vi "Actor Core.vi"(8 "error in":errorcluster, 11 "Nested in":refnum<class "  SEÑAL_ACTUALIZABLE.lvclass">) -> (0 "error out":errorcluster, 3 "Actor out":refnum<class "Actor.lvclass">)   [LabVIEW 2019, in "  SEÑAL_ACTUALIZABLE.lvlib" / "  SEÑAL_ACTUALIZABLE.lvclass"]
doc: "(<B>Filename</B>: Actor Framework.lvlib:Actor.lvclass:Actor Core.vi)\n\nReceives messages to the actor, reacts to them, and initiates any error handling that may shut the actor down.\n\nDescendant classes may override this VI to append parallel tasks for the actor to complete while it handles messages. Overrides use the Call Parent Method node."
uses:
  C:/Program Files (x86)/National Instruments/LabVIEW 2019/vi.lib/ActorFramework/Actor/Actor.lvclass
  <vilib>/ActorFramework/Actor/Actor.lvclass
  GUARDADOTEXTOPLANO/GUARDADOTEXTOPLANO/GUARDADOTEXTOPLANO.lvclass
  <vilib>/ActorFramework/Actor/Actor.lvclass/Actor.ctl
  <vilib>/ActorFramework/Message Enqueuer/Message Enqueuer.lvclass/Message Enqueuer.ctl
  GUARDADOTEXTOPLANO/GUARDADOTEXTOPLANO Messages/SEND_INICIARG Msg/SEND_INICIARG Msg.lvclass/SEND_INICIARG Msg.ctl
  GUARDADOTEXTOPLANO/GUARDADOTEXTOPLANO Messages/DATOS Y GUARDADO Msg/DATOS Y GUARDADO Msg.lvclass/DATOS Y GUARDADO Msg.ctl
  <vilib>/ActorFramework/Message Enqueuer/Init from Existing Queue.vi
  <vilib>/ActorFramework/Message Enqueuer/Enqueue.vi
  <vilib>/ActorFramework/Stop Msg/Stop Msg.lvclass
  C:/Program Files (x86)/National Instruments/LabVIEW 2019/vi.lib/ActorFramework/Message/Message.lvclass
  GUARDADOTEXTOPLANO/GUARDADOTEXTOPLANO Messages/SEND_INICIARG Msg/SEND_INICIARG Msg.lvclass
  GUARDADOTEXTOPLANO/GUARDADOTEXTOPLANO Messages/DATOS Y GUARDADO Msg/DATOS Y GUARDADO Msg.lvclass
  <vilib>/ActorFramework/Message Priority Queue/Priority Enqueue.vi
  <vilib>/ActorFramework/Message Enqueuer/Message Enqueuer.lvclass
panel:
  out "Waveform Graph":waveform(dbl)(graph)
  in  "GUARDAR":bool
  in  "Path 2":path
  in  "Parámetros":T1={"signal type"=enum."Sine Wave", "amplitude"=1.0, "frequency"=10.0} {"frequency" format="%0.2p"; "amplitude" format="%0.2p"}
  in  "EXIT":bool
  in  "STOP":bool
  in  "START":bool
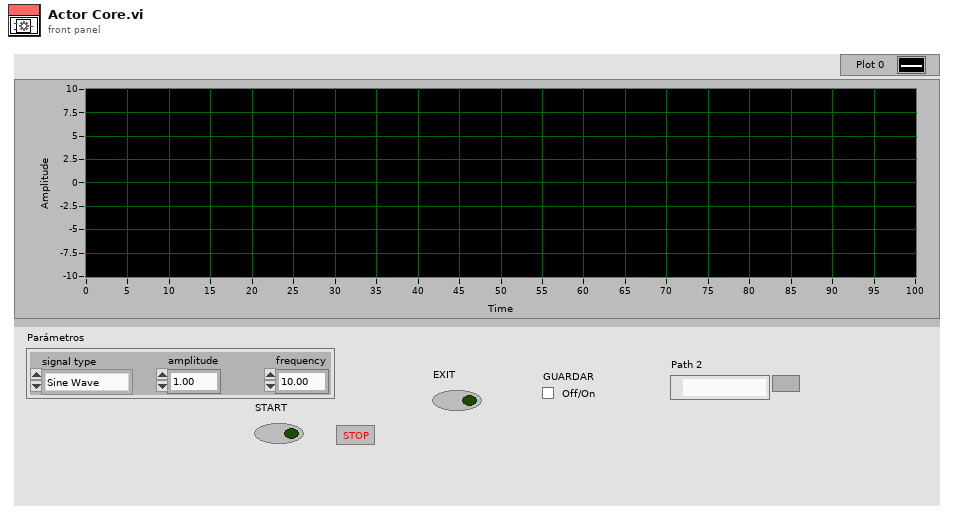
[diagram p1: front panel]
types:
  T1 = cluster{"signal type":enum16{"Sine Wave", "Triangle Wave", "Square Wave", "Sawtooth Wave"}, "amplitude":dbl, "frequency":dbl}
  T2 = cluster{"Stop":refnum<user-event>, "Waveform Graph":refnum<user-event>}
  T3 = enum16{"Sine Wave", "Triangle Wave", "Square Wave", "Sawtooth Wave"}
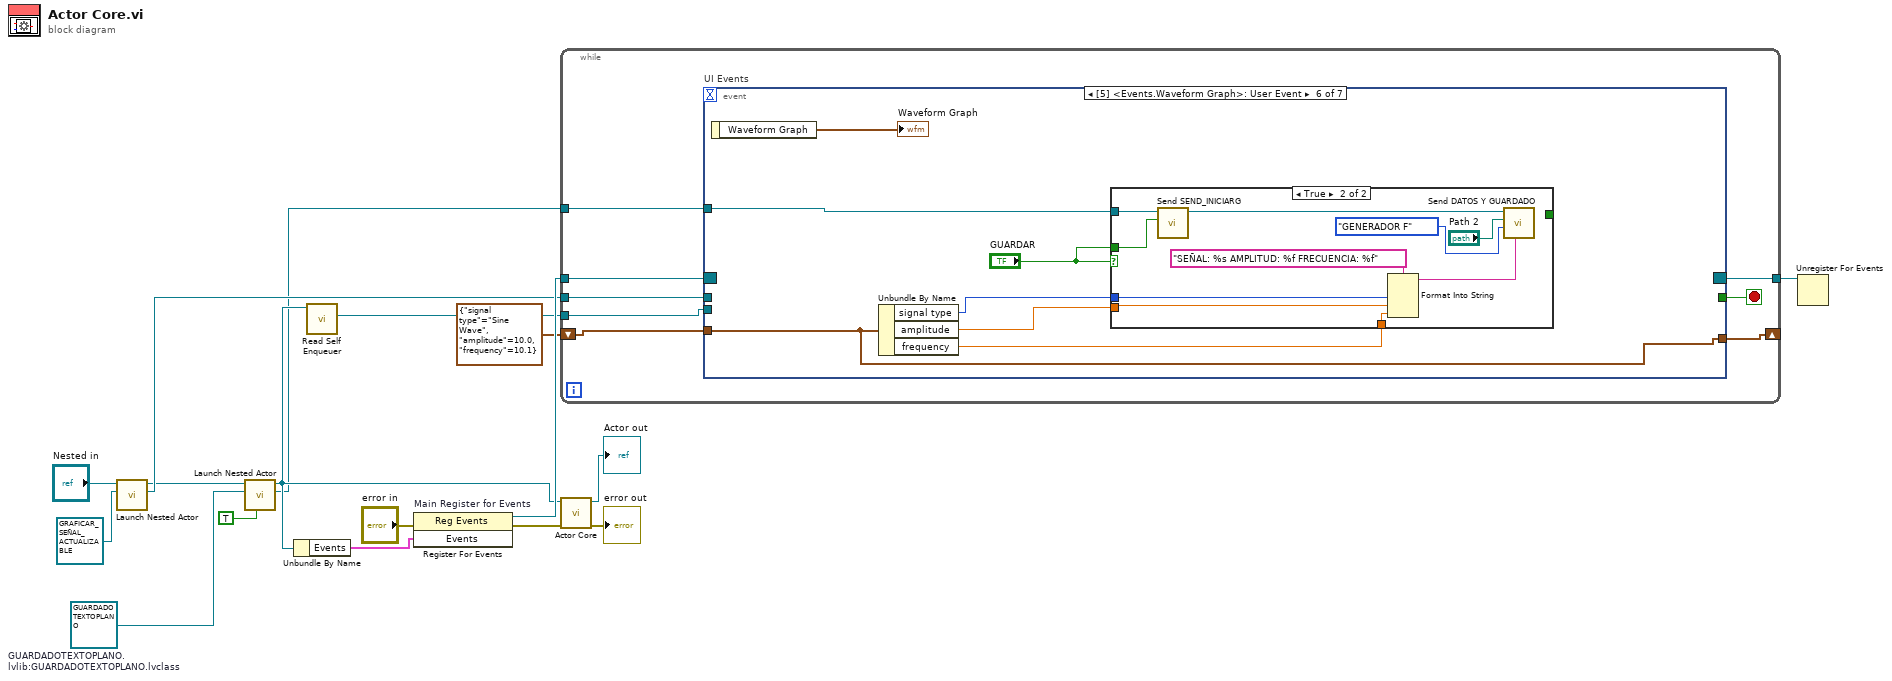
[diagram p0: block diagram]
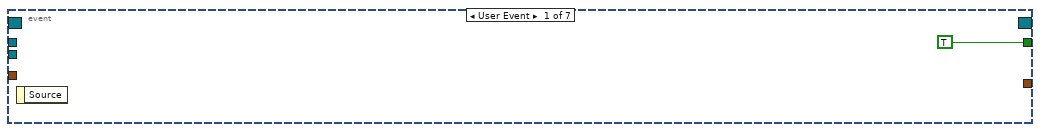
[diagram p2: hidden frame]
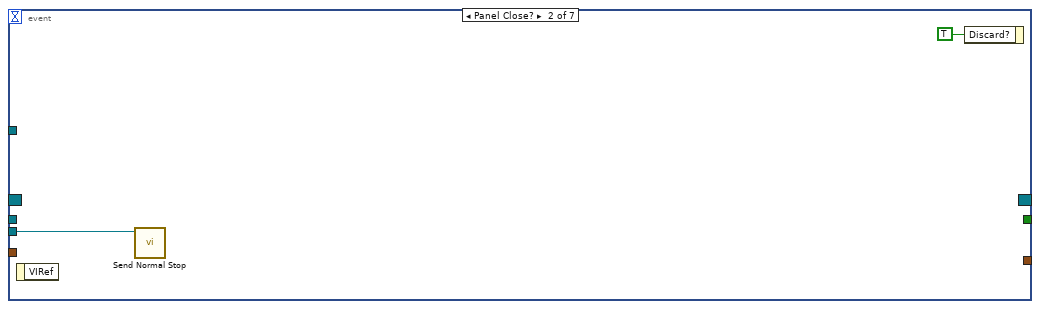
[diagram p3: hidden frame]
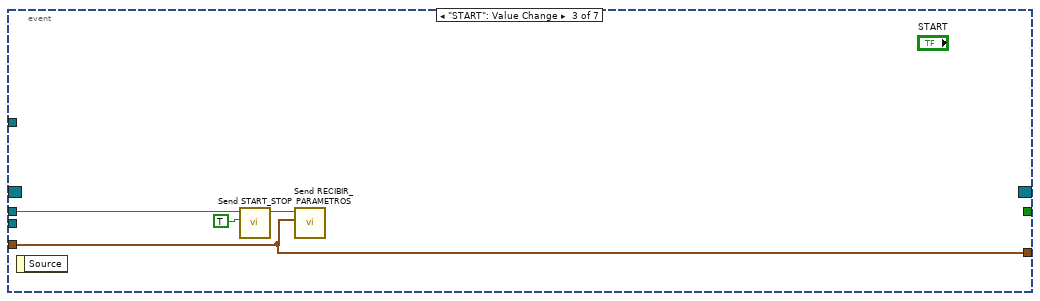
[diagram p4: hidden frame]
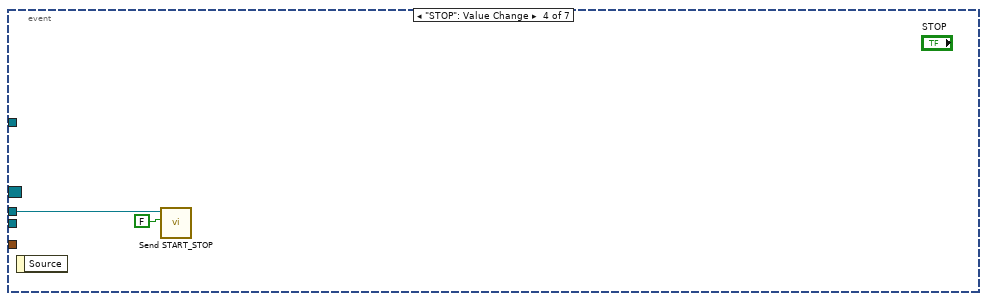
[diagram p5: hidden frame]
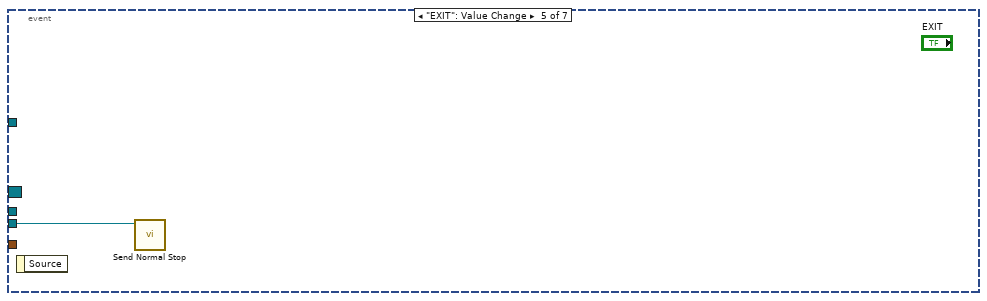
[diagram p6: hidden frame]
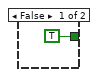
[diagram p7: hidden frame]
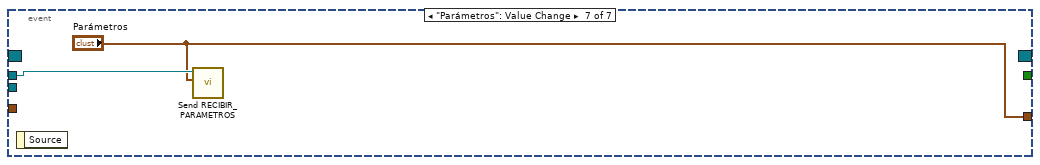
[diagram p8: hidden frame]
diagram:
  w6 = refnum<class "GUARDADOTEXTOPLANO.lvclass"> refnum  # GUARDADOTEXTOPLANO.lvlib:GUARDADOTEXTOPLANO.lvclass
  n1 = call <vilib>:"Launch Nested Actor.vi"("Nested Actor"=refnum<class "GRAFICAR_SEÑAL_ACTUALIZABLE.lvclass"> refnum ("GRAFICAR_SEÑAL_ACTUALIZABLE.lvlib:GRAFICAR_SEÑAL_ACTUALIZABLE.lvclass"), "Caller Actor in"="Nested in") -> ("Nested Actor's Enqueuer"=w8:refnum<class "Message Enqueuer.lvclass">, "Caller Actor out"=w5:refnum<class "  SEÑAL_ACTUALIZABLE.lvclass">)  [unwired: 7 in, 1 out]
  n2 = call <vilib>:"Launch Nested Actor.vi"("Open Actor Core front panel? (F)"=TRUE, "Nested Actor"=w6, "Caller Actor in"=w5) -> ("Nested Actor's Enqueuer"=w3:refnum<class "Message Enqueuer.lvclass">, "Caller Actor out"=w4:refnum<class "  SEÑAL_ACTUALIZABLE.lvclass">)  [unwired: 6 in, 1 out]
  n3 = Unbundle By Name(w4) -> ("Events"=w14:T2)
  n4 = call <vilib>:"Read Self Enqueuer.vi"("Actor"=w4) -> ("Self Enqueuer"=w12:refnum<class "Message Enqueuer.lvclass">)  [unwired: 10 in]
  n5 = register-events "Main Register for Events"(error in="error in", w14) -> (reference out=w15:refnum<event-registration>, error out=w10:errorcluster)  [unwired: 1 in]
  n6 = while {
    tunnel: w15 -> [w25]
    tunnel: [w23] -> w13
    tunnel: w12 -> [w22]
    tunnel: w8 -> [w21]
    tunnel: w3 -> [w20]
    shift-right: [w18] -> _
    shift-left: T1 {"signal type"=enum."Sine Wave", "amplitude"=10.0, "frequency"=10.1} ("Parámetros") -> [w19]
    stop <- w24 stop-if-true
    n7 = event "UI Events" shown="[5] <Events.Waveform Graph>: User Event" {
      selector: w25 -> [_ _ _ _ _ _ _]
      dyn-events: [_ _ _ _ _ _ _] -> w23
      timeout: _ -> [_ _ _ _ _ _ _]
      tunnel: [TRUE _ _ _ _ _ _] -> w24
      tunnel: w22 -> [_ w27 _ _ w35 _ _]
      tunnel: w21 -> [_ _ w32 w34 _ _ w55]
      tunnel: w20 -> [_ _ _ _ _ w42 _]
      tunnel: w19 -> [_ _ w29 _ _ w36 _]
      tunnel: [_ _ w29 _ _ w36 "Parámetros"] -> w18
      event User Event {
        n8 = event-data() -> ()  [unwired: 1 in, 1 out]
      }
      event Panel Close? {
        n9 = event-data() -> ()  [unwired: 1 in, 1 out]
        n10 = call <vilib>:"Send Normal Stop.vi"("Message Enqueuer"=w27) -> ()  [unwired: 10 in, 1 out]
        n11 = event-data("Discard?"=TRUE) -> ()  [unwired: 1 in, 1 out]
      }
      event "START": Value Change {
        n12 = event-data() -> ()  [unwired: 1 in, 1 out]
        n13 = call "Send START_STOP.vi"("START/STOP"=TRUE, "Message Enqueuer"=w32) -> ("Message Enqueuer out"=w30:refnum<class "Message Enqueuer.lvclass">)  [unwired: 8 in, 1 out]
        n14 = call "Send RECIBIR_PARAMETROS.vi"("Parámetros"=w29, "Message Enqueuer"=w30) -> ()  [unwired: 8 in, 2 out]
      }
      event "STOP": Value Change {
        n15 = event-data() -> ()  [unwired: 1 in, 1 out]
        n16 = call "Send START_STOP.vi"("START/STOP"=FALSE, "Message Enqueuer"=w34) -> ()  [unwired: 8 in, 2 out]
      }
      event "EXIT": Value Change {
        n17 = event-data() -> ()  [unwired: 1 in, 1 out]
        n18 = call <vilib>:"Send Normal Stop.vi"("Message Enqueuer"=w35) -> ()  [unwired: 10 in, 1 out]
      }
      event User Event {
        n19 = event-data() -> ("Waveform Graph"=→"Waveform Graph":waveform(dbl))  [unwired: 1 in]
        n20 = Unbundle By Name(w36) -> ("signal type"=w39:T3, "amplitude"=w38:dbl, "frequency"=w37:dbl)
        n21 = case shown="True" "GUARDAR" {
          tunnel: "GUARDAR" -> [_ w53]
          tunnel: w42 -> [_ w49]
          tunnel: [TRUE _] -> _
          tunnel: w39 -> [_ w46]
          tunnel: w38 -> [_ w45]
          tunnel: w37 -> [_ w44]
          frame False {
          }
          frame True {
            n22 = call "Send SEND_INICIARG.vi"("GUARDAR?"=w53, "Message Enqueuer"=w49) -> ("Message Enqueuer out"=w52:refnum<class "Message Enqueuer.lvclass">)  [unwired: 8 in, 1 out]
            n23 = Format Into String(format string="SEÑAL: %s AMPLITUD: %f FRECUENCIA: %f", w46, w45, w44) -> (resulting string=w48:string)  [unwired: 2 in, 1 out]
            n24 = call "Send DATOS Y GUARDADO.vi"("DATO"=w48, "PROVIENE DE?"=enum16{"CONTADOR", "GENERADOR F"}."GENERADOR F", "Path"="Path 2", "Message Enqueuer"=w52) -> ()  [unwired: 6 in, 2 out]
          }
        }
      }
      event "Parámetros": Value Change {
        n25 = event-data() -> ()  [unwired: 1 in, 1 out]
        n26 = call "Send RECIBIR_PARAMETROS.vi"("Parámetros"="Parámetros", "Message Enqueuer"=w55) -> ()  [unwired: 8 in, 2 out]
      }
    }
  }
  n27 = call-parent "Actor Core.vi"("error in"=w10, "Actor in"=w4) -> ("error out"=→"error out":errorcluster, "Actor out"=→"Actor out":refnum<class "Actor.lvclass">)  [unwired: 8 in]
  n28 = Unregister For Events(event registration refnum=w13) -> ()  [unwired: 1 in, 1 out]
